vi "DAQmx计数.vi"() -> ()   [LabVIEW 2010]
uses:
  <vilib>/DAQmx/read.llb/DAQmx Read.vi
  <vilib>/DAQmx/read.llb/DAQmx Read (Counter U32 1Chan 1Samp).vi
  <vilib>/daqmx/miscellaneous.llb/DAQmx Fill In Error Info.vi
panel:
  in  "stop":bool
  out "data":u32
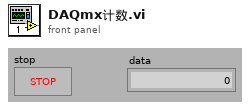
[diagram p1: front panel]
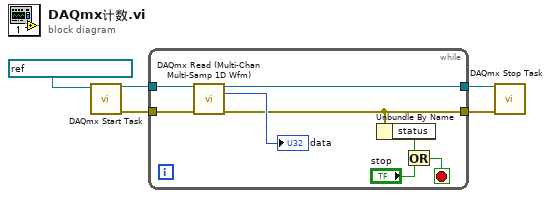
[diagram p0: block diagram]
diagram:
  n1 = call <vilib>:"DAQmx Start Task.vi"("task/channels in"=refnum<k21> "MyCountEdgesTask") -> ("task out"=w5:refnum<k21>, "error out"=w4:errorcluster)  [unwired: 13 in]
  n2 = while {
    tunnel: w5 -> [w13]
    tunnel: w4 -> [w12]
    tunnel: [w8] -> w3
    tunnel: [w11] -> w2
    stop <- w6 stop-if-true
    n3 = call-poly "DAQmx Read (Multi-Chan Multi-Samp 1D Wfm).vi"("task/channels in"=w13, "error in"=w12) -> ("task out"=w11:refnum<k21>, "data"=→"data":u32, "error out"=w8:errorcluster)  [unwired: 11 in]
    n4 = Unbundle By Name(w8) -> ("status"=w9:bool)
    n5 = Or(x=w9, y="stop") -> (x .or. y?=w6:bool)
  }
  n6 = call <vilib>:"DAQmx Stop Task.vi"("task/channels in"=w2, "error in"=w3) -> ()  [unwired: 12 in, 2 out]
